vi "Wait Chart.vi"() -> ()   [LabVIEW 2012]
doc: "This VI is a solution to an exercise in the LabVIEW Core I course.\n\nIt is used to demonstrate the difference between wait functions and elapsed timing."
uses:
  Instance           1 18Saved   Wait Chart .vi
panel:
  out "Chart 2":dbl(graph)
  out "Chart 1":dbl(graph)
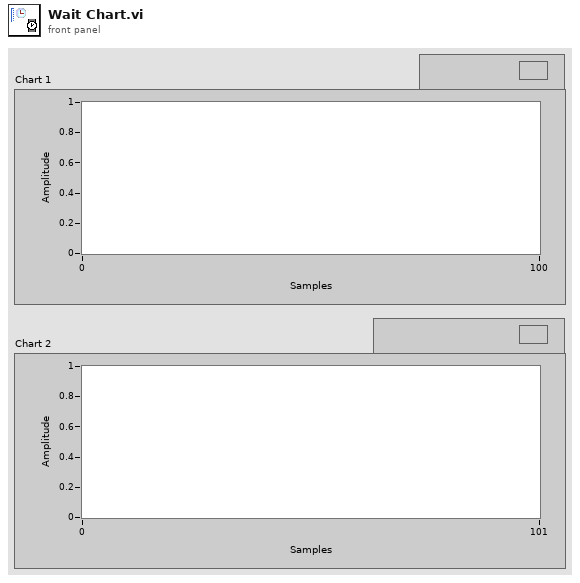
[diagram p1: front panel]
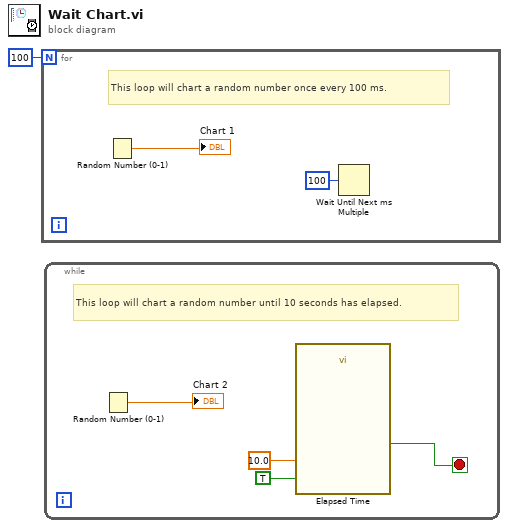
[diagram p0: block diagram]
diagram:
  n1 = for {
    N: 100 -> [_]
    # "This loop will chart a random number once every 100 ms."
    n2 = Random Number (0-1)() -> (number: 0 to 1=→"Chart 1":dbl)
    n3 = Wait Until Next ms Multiple(millisecond multiple=u32 100) -> ()  [unwired: 1 out]
  }
  n4 = while {
    stop <- w7 stop-if-true
    # "This loop will chart a random number until 10 seconds has elapsed."
    n5 = Random Number (0-1)() -> (number: 0 to 1=→"Chart 2":dbl)
    n6 = call "Elapsed Time"("Time Target (s)"=10.0, "Auto Reset"=TRUE) -> ("Time has Elapsed"=w7:bool)  [unwired: 10 in, 7 out]
  }
